vi "Write_para_port0.vi"(8 "error in (no error)":errorcluster caption="错误输入（无错误）", 10 "port0（8元素）":bool[](array[boolean]), 11 "address":i16=888 caption="地址" format="%.0x") -> (0 "error out":errorcluster caption="错误输出")   [LabVIEW 2011]
uses:
  <vilib>/Platform/portaccess.llb/Out Port8.vi
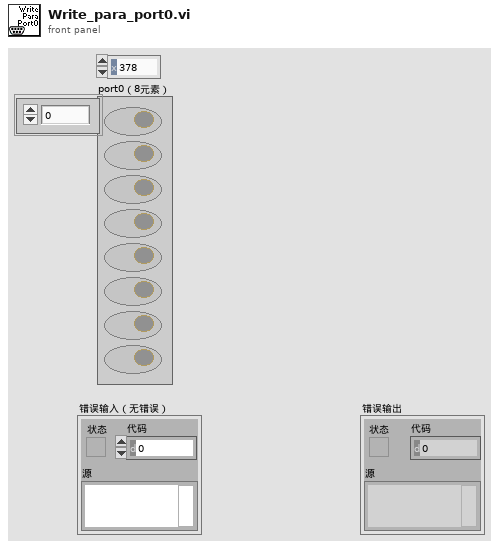
[diagram p1: front panel]
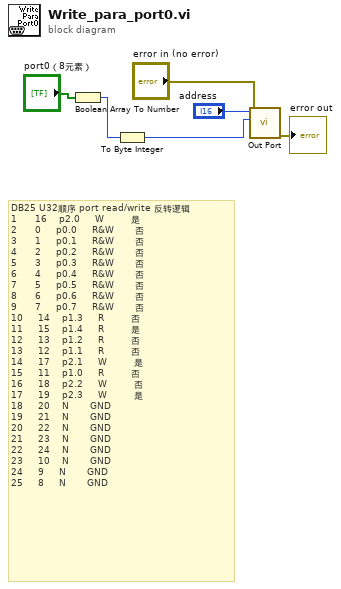
[diagram p0: block diagram]
diagram:
  # "DB25\tU32顺序\tport\tread/write\t反转逻辑\n1\t     16\t   p2.0    \tW\t        是\n2\t     0    \tp0.0\t   \tR&W\t      否\n3\t     1\t\t   p0.1\t   \tR&W      \t否\n4\t\t    2\t   \tp0.2   \t\tR&W      \t否\n5\t\t    3\t\t   p0.3   \t\tR&W\t      否\n6\t\t    4\t   \tp0.4   \t\tR&W      \t否\n7\t\t    5\t   \tp0.5   \t\tR&W      \t否\n8\t\t    6\t   \tp0.6\t   \tR&W      \t否\n9\t    \t7\t   \tp0.7\t   \tR&W\t      否\n10\t    14   \tp1.3   \t\tR        \t否\n11\t   \t15   \tp1.4   \t\tR        \t是\n12\t   \t13   \tp1.2\t   \tR        \t否\n13    \t12   \tp1.1\t   \tR        \t否\n14     17   \tp2.1\t   \tW        \t是\n15    \t11   \tp1.0   \t\tR\t        否\n16    \t18   \tp2.2   \t\tW        \t否\n17    \t19\t   p2.3   \t\tW\t        是\n18    \t20   \tN   \t  \tGND\t\n19    \t21   \tN   \t  \tGND\t\n20\t    22\t   N\t  \t  \tGND\t\n21\t    23\t   N  \t  \t\tGND\t\n22\t    24\t   N  \t  \t\tGND\t\n23    \t10   \tN  \t  \t\tGND\t\n24    \t9\t    N  \t  \t\tGND\t\n25\t    8    \tN  \t  \t\tGND"
  n1 = Boolean Array To Number(Boolean array="port0（8元素）") -> (number=w2:u32)
  n2 = To Byte Integer(number=w2) -> (8bit integer=w1:i8)
  n3 = call-poly <vilib>:"Out Port.vi"("error in (no error)"="error in (no error)", "write value"=w1, "address"="address") -> ("error out"=→"error out":errorcluster)  [unwired: 6 in]
